vi "gaussianIntensityImage.vi"(5 "stdNoise":dbl, 6 "range":dbl=1.0, 7 "nbits":u32=12, 8 "rows":i32=11, 9 "cols":i32=11, 10 "y pars":dbl[](array[numeric])=[1.0, 5.0, 3.0, 0.0], 11 "x pars":dbl[](array[numeric])=[1.0, 5.0, 3.0, 0.0]) -> (3 "Intesity":u32[][](array[numeric]))   [LabVIEW 2021]
uses:
  <vilib>/Analysis/NI_AALBase.lvlib
panel:
  in  "offset":i32
  out "max intesisty":u32
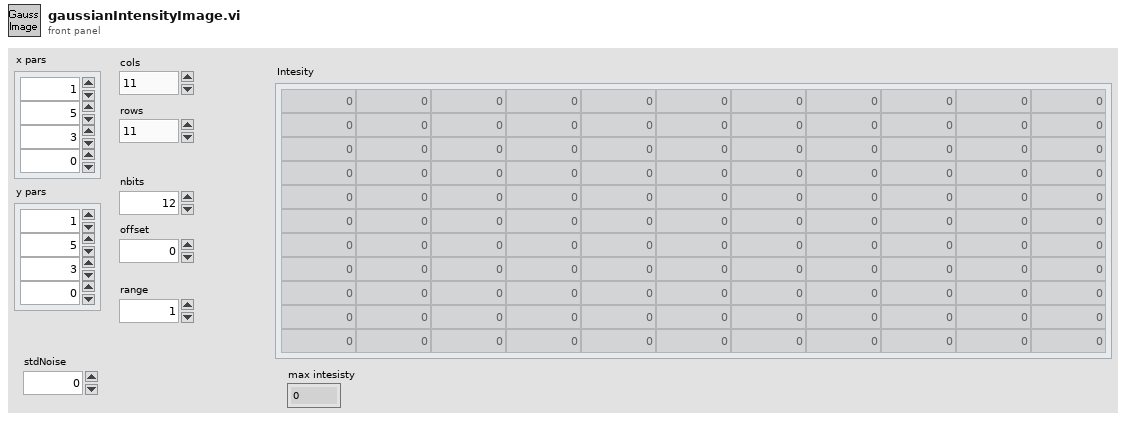
[diagram p1: front panel]
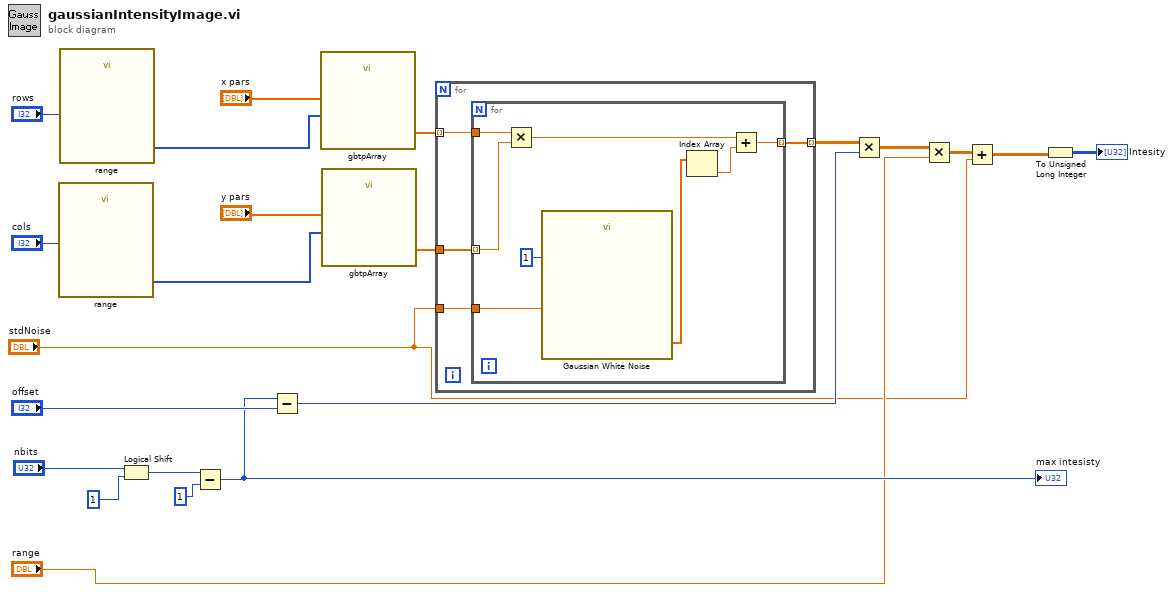
[diagram p0: block diagram]
diagram:
  n1 = call "range.vi"("end"="cols") -> ("range"=w14:i32[])  [unwired: 10 in]
  n2 = call "range.vi"("end"="rows") -> ("range"=w17:i32[])  [unwired: 10 in]
  n3 = Logical Shift(y="nbits", x=1 ("x << y")) -> (x << y=w11:i32)
  n4 = Subtract(x=w11, y=1) -> (x-y=w8:i32)
  "max intesisty" <- w8
  n5 = Subtract(x=w8, y="offset") -> (x-y=w7:i32)
  n6 = call "gbtpArray.vi"("X"=w17, "P"="x pars") -> ("f(X;P)"=w20:dbl[])
  n7 = call "gbtpArray.vi"("X"=w14, "P"="y pars") -> ("f(X;P)"=w19:dbl[])
  n8 = for {
    tunnel: w20 -> [w26] mode=indexing
    tunnel: w19 -> [w25]
    tunnel: [w24] -> w5 mode=indexing
    tunnel: "stdNoise" -> [w23]
    n9 = for {
      tunnel: w26 -> [w34]
      tunnel: w25 -> [w33] mode=indexing
      tunnel: [w31] -> w24 mode=indexing
      tunnel: w23 -> [w30]
      n10 = Multiply(x=w34, y=w33) -> (x*y=w32:dbl)
      n11 = call <vilib>:"Gaussian White Noise.vi"("standard deviation"=w30, "samples"=1) -> ("Gaussian noise pattern"=w28:dbl[])  [unwired: 8 in, 1 out]
      n12 = Index Array(array=w28) -> (element=w27:dbl)  [unwired: 1 in]
      n13 = Add(x=w32, y=w27) -> (x+y=w31:dbl)
    }
  }
  n14 = Multiply(x=w5, y=w7) -> (x*y=w18:dbl[][])
  n15 = Multiply(x=w18, y="range") -> (x*y=w3:dbl[][])
  n16 = Add(x=w3, y="stdNoise") -> (x+y=w2:dbl[][])
  n17 = To Unsigned Long Integer(number=w2) -> (unsigned 32bit integer=→"Intesity":u32[][])
